vi "Write Settings.vi"(8 "error in (no error)":errorcluster, 10 "Settings 2":T1, 11 "FakeCamera in":refnum<class "MoveDataFile.lvclass">) -> (0 "error out":errorcluster, 3 "FakeCamera out":refnum<class "MoveDataFile.lvclass">)   [LabVIEW 2011, in "MoveDataFile.lvclass"]
uses:
  MoveDataFile.lvclass
  SettingsTypdef.ctl
  shared/OnOffTypeDef.ctl
  MoveDataFile.lvclass/MoveDataFile.ctl
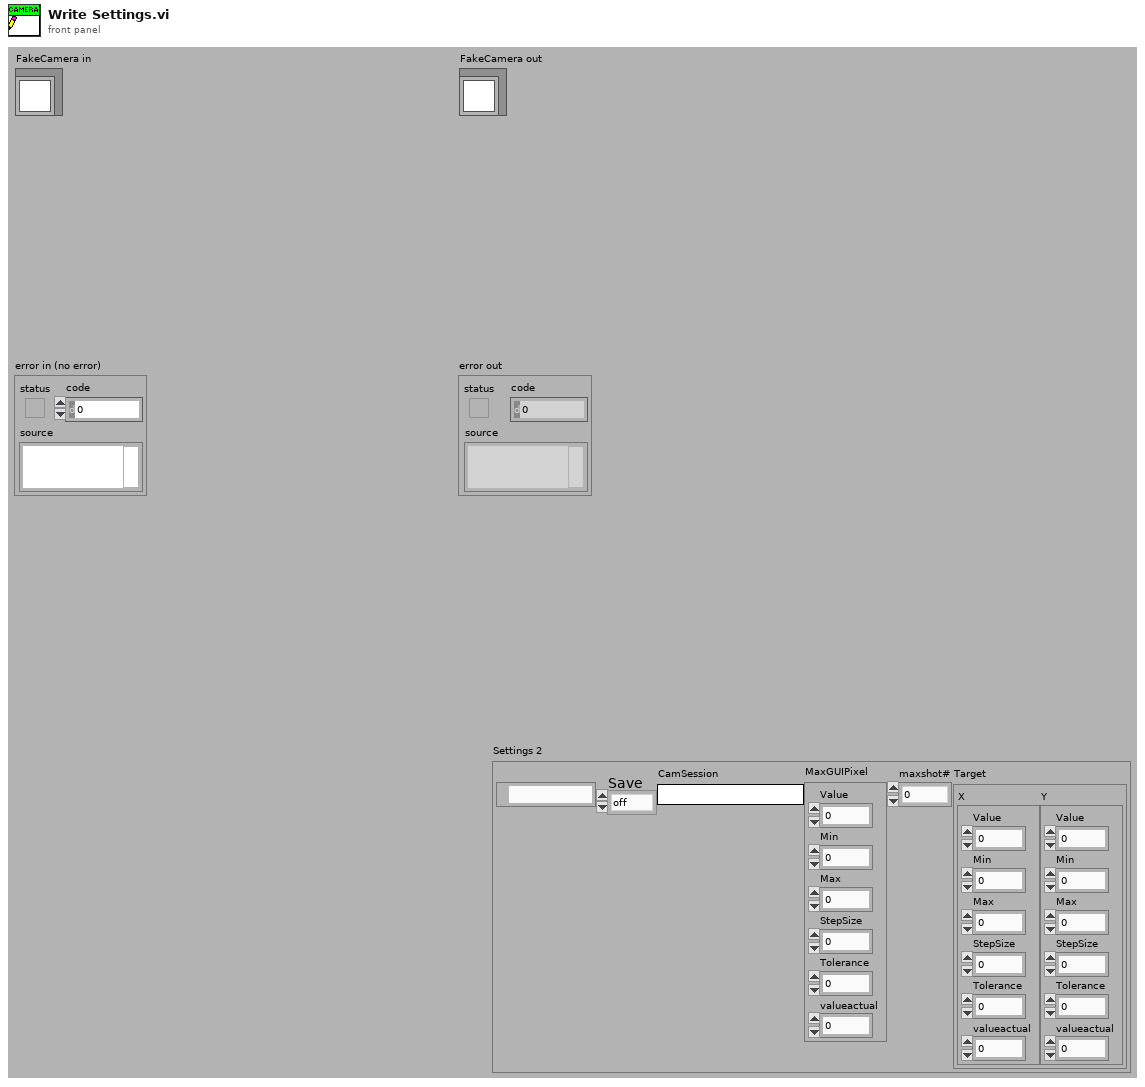
[diagram p1: front panel]
types:
  T1 = typedef "MoveDataFile.lvclass/SettingsTypdef.ctl" = cluster{"LocalSavingPath":path, "Save":T2, "CamSession":string, "MaxGUIPixel":cluster{"Value":dbl, "Min":dbl, "Max":dbl, "StepSize":dbl, "Tolerance":dbl, "valueactual":dbl}, "maxshot#":dbl, "Target":cluster{"X":cluster{"Value":dbl, "Min":dbl, "Max":dbl, "StepSize":dbl, "Tolerance":dbl, "valueactual":dbl}, "Y":cluster{"Value":dbl, "Min":dbl, "Max":dbl, "StepSize":dbl, "Tolerance":dbl, "valueactual":dbl}}}
  T2 = typedef "OnOffTypeDef.ctl" = enum16{"off", "on"}
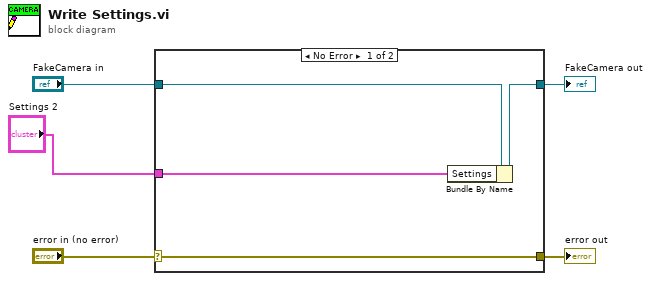
[diagram p0: block diagram]
diagram:
  n1 = case shown="No Error" "error in (no error)" {
    selector: "error in (no error)" -> [w9 w10]
    tunnel: [w9 w10] -> w4
    tunnel: [w7 w11] -> w2
    tunnel: "FakeCamera in" -> [w8 w11]
    tunnel: "Settings 2" -> [w6 _]
    frame No Error {
      n2 = Bundle By Name(cluster=w8, "Settings"=w6) -> (w7:refnum<class "MoveDataFile.lvclass">)
    }
    frame Error {
    }
  }
  "error out" <- w4
  "FakeCamera out" <- w2
